vi "VisualizeStatus.vi"(10 "ModuleList":string[](array[string])=["Sync", "FGen", "Digitizer", "Sensor", "Analysis", "Scope", "AcPwr"]) -> ()   [LabVIEW 2018, in "Visualization.lvlib" / "VisualizeStatus.lvclass"]
uses:
  VisualizeStatus.lvclass
  <vilib>/event_ctls.llb/usereventprio.ctl
  VisualizeBase/VisualizeBase_class/Requests/clUserEventType.ctl
  <vilib>/Utility/error.llb/Error Cluster From Error Code.vi
  <vilib>/ErrorRing/Error Ring.xnode
  VisualizeBase/VisualizeBase_class/VisualizeBase.lvclass
  <userlib>/NIST/NISTErrorLib/NISTErrorLib.lvlib
  Sync/SyncModule/SyncModule.lvlib
  Digitizer/DigitizerModule/DigitizerModule.lvlib
  FGen/FgenModule/FgenModule.lvlib
  BusClass/Bus.lvclass
  Sensor/SensorModule/SensorModule.lvlib
  Analysis/AnalysisModule/AnalysisModule.lvlib
  Scope/ScopeModule/ScopeModule.lvlib
panel:
  out "Status Message":string
  in  "btnReset":bool
  in  "btnClear":bool
  in  "QueName":string="BaseVisQue"
  out "ErrorArray":errorcluster[](array[cluster])
  in  "btnStop":bool
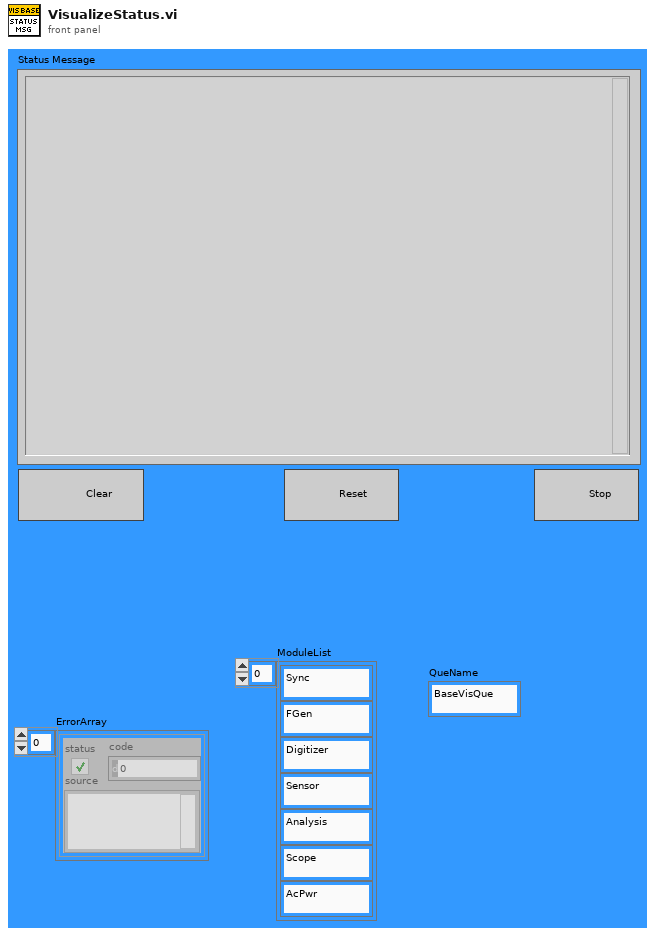
[diagram p1: front panel]
types:
  T1 = typedef "SyncModule.lvlib/clBroadcastEvents.ctl" = cluster{"DidInit":refnum<user-event>, "StatusUpdate":refnum<user-event>, "ErrorReport":refnum<user-event>, "DidStop":refnum<user-event>, "PathToINI":refnum<user-event>, "TriggerTime":refnum<user-event>, "LockStatus":refnum<user-event>, "Info":refnum<user-event>, "ClockProperties":refnum<user-event>}
  T2 = typedef "FgenModule.lvlib/clBroadcastEvents.ctl" = cluster{"DidInit":refnum<user-event>, "StatusUpdate":refnum<user-event>, "ErrorReport":refnum<user-event>, "DidStop":refnum<user-event>, "PathToINI":refnum<user-event>, "Channels":refnum<user-event>, "Function":refnum<user-event>, "Waveforms":refnum<user-event>, "Triggers":refnum<user-event>, "FunctionParams":refnum<user-event>, "FunctionArbs":refnum<user-event>, "FunctionSampleRate":refnum<user-event>}
  T3 = typedef "ScopeModule.lvlib/clBroadcastEvents.ctl" = cluster{"DidInit":refnum<user-event>, "StatusUpdate":refnum<user-event>, "ErrorReport":refnum<user-event>, "DidStop":refnum<user-event>, "PathToINI":refnum<user-event>, "Handle":refnum<user-event>, "Model":refnum<user-event>, "Channels":refnum<user-event>, "Acquisition":refnum<user-event>, "Trigger":refnum<user-event>, "ExtAcquisition":refnum<user-event>, "Waveform":refnum<user-event>}
  T4 = typedef "DigitizerModule.lvlib/clBroadcastEvents.ctl" = cluster{"DidInit":refnum<user-event>, "StatusUpdate":refnum<user-event>, "ErrorReport":refnum<user-event>, "DidStop":refnum<user-event>, "PathToINI":refnum<user-event>, "Channels":refnum<user-event>, "Acq":refnum<user-event>, "Trigger":refnum<user-event>, "Waveforms":refnum<user-event>}
  T5 = typedef "SensorModule.lvlib/clBroadcastEvents.ctl" = cluster{"DidInit":refnum<user-event>, "StatusUpdate":refnum<user-event>, "ErrorReport":refnum<user-event>, "DidStop":refnum<user-event>, "PathToINI":refnum<user-event>, "SensorReport":refnum<user-event>, "SensorConfig":refnum<user-event>}
  T6 = typedef "AnalysisModule.lvlib/clBroadcastEvents.ctl" = cluster{"DidInit":refnum<user-event>, "StatusUpdate":refnum<user-event>, "ErrorReport":refnum<user-event>, "DidStop":refnum<user-event>, "PathToINI":refnum<user-event>, "Config":refnum<user-event>, "ResultReport":refnum<user-event>, "FunctionClass":refnum<user-event>, "State":refnum<user-event>, "FunctionParams":refnum<user-event>}
  T7 = typedef "clBroadcastEvents.ctl" = cluster{"DidInit":refnum<user-event>, "StatusUpdate":refnum<user-event>, "ErrorReport":refnum<user-event>, "DidStop":refnum<user-event>, "PathToINI":refnum<user-event>, "Measurements":refnum<user-event>, "LoadConfigFile":refnum<user-event>, "GetSettings":refnum<user-event>, "SetSettings":refnum<user-event>, "GetType&ID":refnum<user-event>, "GotSettings":refnum<user-event>}
  T8 = cluster{"StatusUpdate":refnum<user-event>, "ErrorReport":refnum<user-event>}
  T9 = typedef "Visualization.lvlib/VisualizeBase.lvclass/clRequestEvents.ctl" = cluster{"StopRequest":refnum<user-event>, "ResetRequest":refnum<user-event>}
  T10 = typedef "usereventprio.ctl" = enum32{"high priority", "normal priority"}
  T11 = typedef "Visualization.lvlib/VisualizeBase.lvclass/clUserEventType.ctl" = cluster{"BusIndex":i8, "Data":variant}
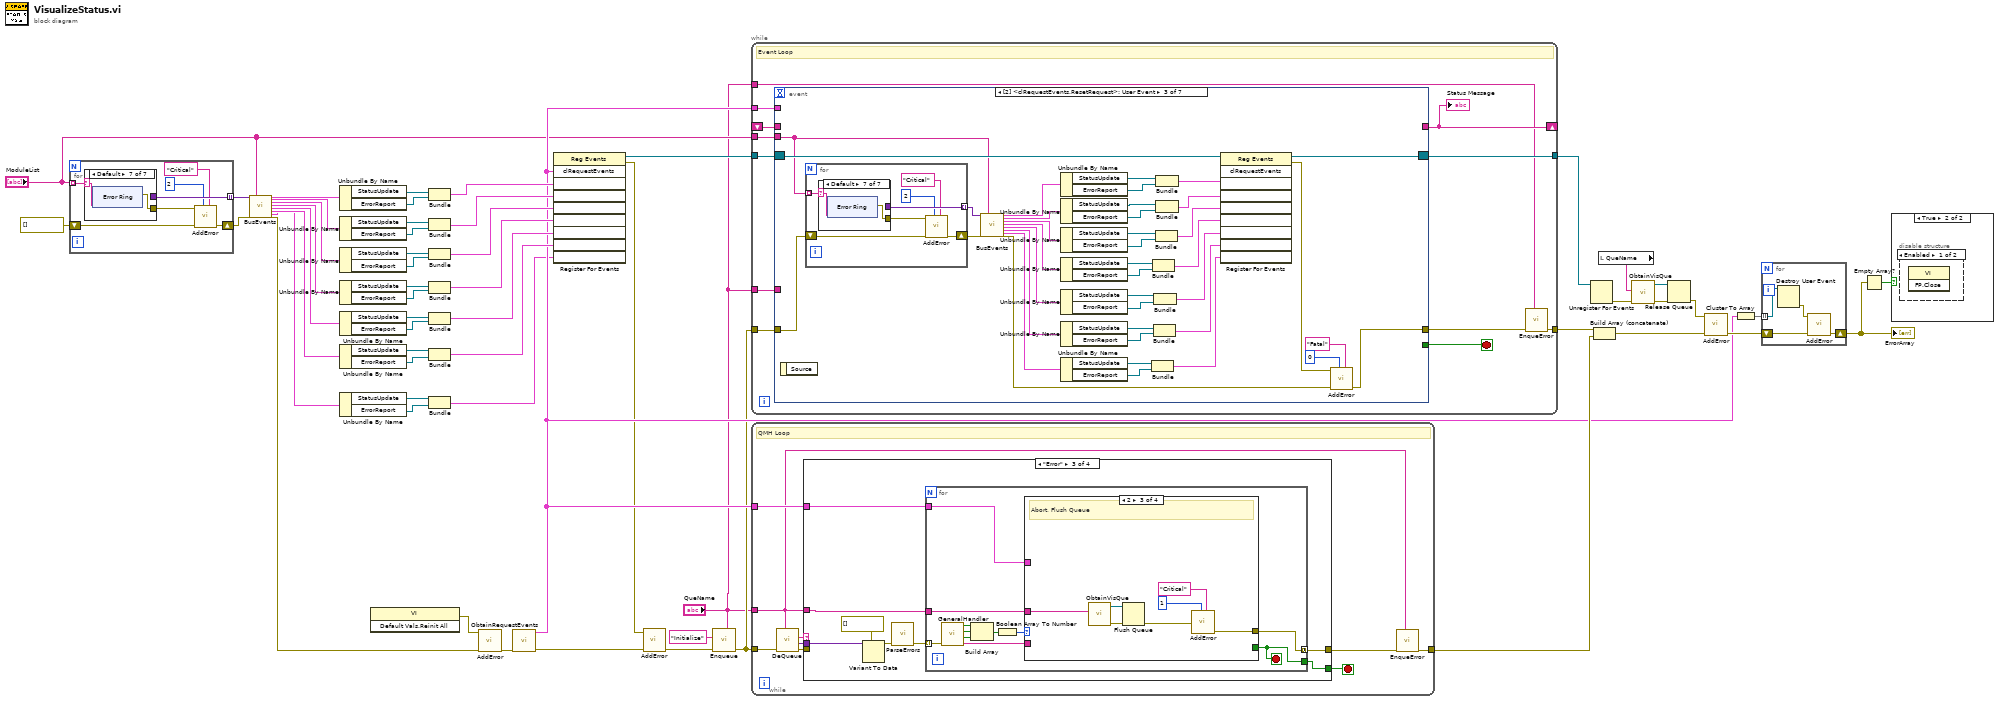
[diagram p0: block diagram]
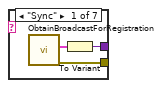
[diagram p2: hidden frame]
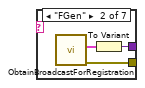
[diagram p3: hidden frame]
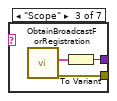
[diagram p4: hidden frame]
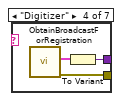
[diagram p5: hidden frame]
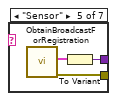
[diagram p6: hidden frame]
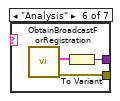
[diagram p7: hidden frame]
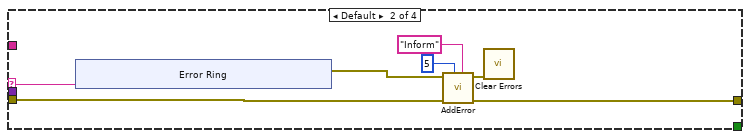
[diagram p9: hidden frame]
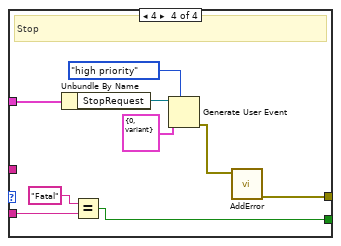
[diagram p12: hidden frame]
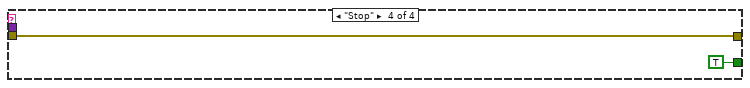
[diagram p13: hidden frame]
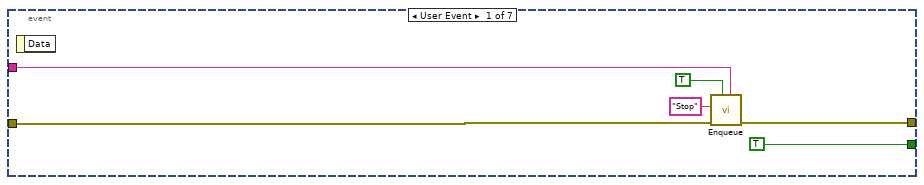
[diagram p14: hidden frame]
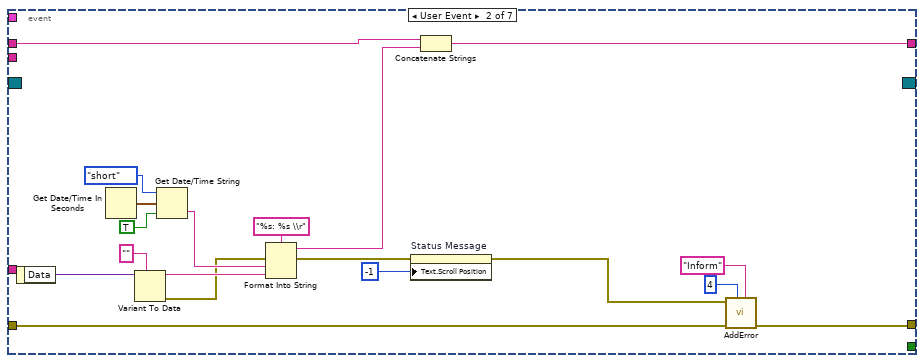
[diagram p15: hidden frame]
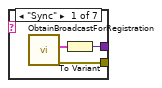
[diagram p16: hidden frame]
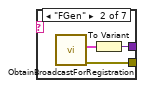
[diagram p17: hidden frame]
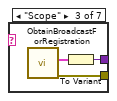
[diagram p18: hidden frame]
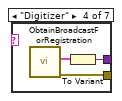
[diagram p19: hidden frame]
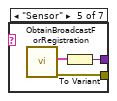
[diagram p20: hidden frame]
diagram:
  n1 = for {
    shift-right: [w62] -> w22
    shift-left: errorcluster[] [] ("ErrorArray") -> [w61]
    tunnel: [w60] -> w23 mode=indexing
    tunnel: "ModuleList" -> [w57] mode=indexing
    n2 = case shown="Default" w57 {
      selector: w57 -> [_ _ _ _ _ _ w82]
      tunnel: [w65 w68 w70 w74 w77 w80 _] -> w60
      tunnel: [w64 w69 w72 w75 w78 w81 w83] -> w63
      frame "Sync" {
        n3 = call "ObtainBroadcastForRegistration.vi"() -> ("error out"=w64:errorcluster, "SyncBroadcastEvents"=w66:T1)  [unwired: 10 in]
        n4 = To Variant(anything=w66) -> (Variant=w65:variant)
      }
      frame "FGen" {
        n5 = call "ObtainBroadcastForRegistration.vi"() -> ("error out"=w69:errorcluster, "clBroadcastEvents"=w67:T2)  [unwired: 10 in]
        n6 = To Variant(anything=w67) -> (Variant=w68:variant)
      }
      frame "Scope" {
        n7 = call "ObtainBroadcastForRegistration.vi"() -> ("error out"=w72:errorcluster, "clBroadcastEvents"=w71:T3)  [unwired: 10 in]
        n8 = To Variant(anything=w71) -> (Variant=w70:variant)
      }
      frame "Digitizer" {
        n9 = call "ObtainBroadcastForRegistration.vi"() -> ("error out"=w75:errorcluster, "clDigitizerBdcstEvents"=w73:T4)  [unwired: 10 in]
        n10 = To Variant(anything=w73) -> (Variant=w74:variant)
      }
      frame "Sensor" {
        n11 = call "ObtainBroadcastForRegistration.vi"() -> ("error out"=w78:errorcluster, "SensorBdcstEvents"=w76:T5)  [unwired: 10 in]
        n12 = To Variant(anything=w76) -> (Variant=w77:variant)
      }
      frame "Analysis" {
        n13 = call "ObtainBroadcastForRegistration.vi"() -> ("error out"=w81:errorcluster, "AnalysisBroadcastEvents"=w79:T6)  [unwired: 10 in]
        n14 = To Variant(anything=w79) -> (Variant=w80:variant)
      }
      frame Default {
        n15 = xnode "Error Ring"("parameter 0"=w82) -> ("error out"=w83:errorcluster)
      }
    }
    n16 = call <userlib>:"AddError.vi"("Severity"="Critical", "Priority"=u8 2, "ErrorArray"=w61, "error in (no error)"=w63) -> ("ErrorArray"=w62:errorcluster[])  [unwired: 6 in, 1 out]
  }
  n17 = call "BusEvents.vi"("EventArray"=w23, "Error in"=w22, "ModuleList"="ModuleList") -> ("SyncEvts"=w32:T1, "FGenEvts"=w31:T2, "DigitizerEvts"=w30:T4, "AnalysisBroadcastEvents"=w25:T6, "SensorBdcstEvents"=w24:T5, "ScopeBdcstEvents"=w16:T3, "clAcPwrEvents"=w5:T7, "Error out"=w6:errorcluster[])  [unwired: 16 in, 1 out]
  n18 = Unbundle By Name(w32) -> ("StatusUpdate"=w39:refnum<user-event>, "ErrorReport"=w38:refnum<user-event>)
  n19 = Unbundle By Name(w31) -> ("StatusUpdate"=w37:refnum<user-event>, "ErrorReport"=w36:refnum<user-event>)
  n20 = Unbundle By Name(w30) -> ("StatusUpdate"=w35:refnum<user-event>, "ErrorReport"=w34:refnum<user-event>)
  n21 = Unbundle By Name(w25) -> ("StatusUpdate"=w28:refnum<user-event>, "ErrorReport"=w29:refnum<user-event>)
  n22 = Unbundle By Name(w24) -> ("StatusUpdate"=w27:refnum<user-event>, "ErrorReport"=w26:refnum<user-event>)
  n23 = Unbundle By Name(w16) -> ("StatusUpdate"=w18:refnum<user-event>, "ErrorReport"=w17:refnum<user-event>)
  n24 = Unbundle By Name(w5) -> ("StatusUpdate"=w8:refnum<user-event>, "ErrorReport"=w9:refnum<user-event>)
  n25 = invoke class="VI" method="Default Vals.Reinit All"() -> (error out=w55:errorcluster)  [unwired: 3 in, 2 out]
  n26 = Bundle("StatusUpdate"=w39, "ErrorReport"=w38) -> (w15:T8)  [unwired: 1 in]
  n27 = Bundle("StatusUpdate"=w37, "ErrorReport"=w36) -> (w13:T8)  [unwired: 1 in]
  n28 = Bundle("StatusUpdate"=w35, "ErrorReport"=w34) -> (w14:T8)  [unwired: 1 in]
  n29 = Bundle("StatusUpdate"=w28, "ErrorReport"=w29) -> (w12:T8)  [unwired: 1 in]
  n30 = Bundle("StatusUpdate"=w27, "ErrorReport"=w26) -> (w20:T8)  [unwired: 1 in]
  n31 = Bundle("StatusUpdate"=w18, "ErrorReport"=w17) -> (w19:T8)  [unwired: 1 in]
  n32 = Bundle("StatusUpdate"=w8, "ErrorReport"=w9) -> (w7:T8)  [unwired: 1 in]
  n33 = call <userlib>:"AddError.vi"("ErrorArray"=w6, "error in (no error)"=w55) -> ("ErrorArray"=w54:errorcluster[])  [unwired: 8 in, 1 out]
  n34 = call "ObtainRequestEvents.vi"("Error"=w54) -> ("Error"=w53:errorcluster[], "clRequestEvents"=w11:T9)  [unwired: 9 in]
  n35 = register-events(w11, w15, w13, w14, w12, w20, w19, w7) -> (reference out=w21:refnum<event-registration>, error out=w10:errorcluster)  [unwired: 2 in]
  n36 = call <userlib>:"AddError.vi"("ErrorArray"=w53, "error in (no error)"=w10) -> ("ErrorArray"=w33:errorcluster[])  [unwired: 8 in, 1 out]
  n37 = call "Enqueue.vi"("QueName"="QueName", "Error"=w33, "Message"="Initialize") -> ("Error"=w3:errorcluster[])  [unwired: 8 in]
  n38 = while {
    tunnel: w21 -> [w102]
    tunnel: [w99] -> w50
    tunnel: [w98] -> w52
    tunnel: w11 -> [w97]
    shift-right: [w93] -> _
    shift-left: _ -> [w96]
    tunnel: w3 -> [w95]
    tunnel: "ModuleList" -> [w94]
    tunnel: "QueName" -> [w92]
    tunnel: "QueName" -> [w91]
    stop <- w101 stop-if-true
    # "Event Loop"
    n39 = event shown="[2] <clRequestEvents.ResetRequest>: User Event" {
      selector: w102 -> [_ _ w143 _ _ _ _]
      dyn-events: [_ _ w145 _ _ _ _] -> w98
      timeout: _ -> [_ _ _ _ _ _ _]
      tunnel: [TRUE _ _ _ _ _ _] -> w101
      tunnel: [w107 w118 w160 w210 _ w228 w233] -> w100
      tunnel: w97 -> [_ _ _ _ _ w223 w232]
      tunnel: [_ w114 _ w205 "" _ _] -> w93
      tunnel: w96 -> [_ w113 _ w204 _ _ _]
      tunnel: w95 -> [w103 w112 w138 w201 _ w222 w231]
      tunnel: w94 -> [_ _ w137 _ _ _ _]
      tunnel: w91 -> [w104 _ _ _ _ _ _]
      event User Event {
        n40 = event-data() -> ()  [unwired: 1 in, 1 out]
        n41 = call "Enqueue.vi"("QueName"=w104, "Priority? (F)"=TRUE, "Error"=w103, "Message"="Stop") -> ("Error"=w107:errorcluster[])  [unwired: 7 in]
      }
      event User Event {
        n42 = event-data() -> ("Data"=w124:variant)  [unwired: 1 in]
        n43 = Get Date/Time In Seconds() -> (seconds since 1Jan1904=w127:timestamp)
        n44 = Variant To Data(type="", Variant=w124) -> (data=w120:string, error out=w119:errorcluster)  [unwired: 1 in]
        n45 = Get Date/Time String(date format (0)=enum16{"short", "long", "abbreviated"}."short", seconds (now)=w127, want seconds? (F)=TRUE) -> (time string=w121:string)  [unwired: 1 out]
        n46 = Format Into String(format string="%s: %s \\r", error in=w119, w121, w120) -> (resulting string=w115:string, error out=w111:errorcluster)  [unwired: 1 in]
        n47 = property on="Status Message" class="Str"(error in=w111, "Text.Scroll Position"=-1) -> (error out=w110:errorcluster)  [unwired: 1 in, 1 out]
        n48 = Concatenate Strings(w113, w115) -> (w114:string)
        n49 = call <userlib>:"AddError.vi"("Severity"="Inform", "Priority"=u8 4, "ErrorArray"=w112, "error in (no error)"=w110) -> ("ErrorArray"=w118:errorcluster[])  [unwired: 6 in, 1 out]
      }
      event User Event {
        n50 = event-data() -> ()  [unwired: 1 in, 1 out]
        n51 = for {
          shift-right: [w172] -> w148
          shift-left: w138 -> [w171]
          tunnel: [w170] -> w146 mode=indexing
          tunnel: w137 -> [w167] mode=indexing
          n52 = case shown="Default" w167 {
            selector: w167 -> [_ _ _ _ _ _ w192]
            tunnel: [w175 w178 w182 w184 w187 w190 _] -> w170
            tunnel: [w174 w179 w181 w185 w188 w191 w193] -> w173
            frame "Sync" {
              n53 = call "ObtainBroadcastForRegistration.vi"() -> ("error out"=w174:errorcluster, "SyncBroadcastEvents"=w176:T1)  [unwired: 10 in]
              n54 = To Variant(anything=w176) -> (Variant=w175:variant)
            }
            frame "FGen" {
              n55 = call "ObtainBroadcastForRegistration.vi"() -> ("error out"=w179:errorcluster, "clBroadcastEvents"=w177:T2)  [unwired: 10 in]
              n56 = To Variant(anything=w177) -> (Variant=w178:variant)
            }
            frame "Scope" {
              n57 = call "ObtainBroadcastForRegistration.vi"() -> ("error out"=w181:errorcluster, "clBroadcastEvents"=w180:T3)  [unwired: 10 in]
              n58 = To Variant(anything=w180) -> (Variant=w182:variant)
            }
            frame "Digitizer" {
              n59 = call "ObtainBroadcastForRegistration.vi"() -> ("error out"=w185:errorcluster, "clDigitizerBdcstEvents"=w183:T4)  [unwired: 10 in]
              n60 = To Variant(anything=w183) -> (Variant=w184:variant)
            }
            frame "Sensor" {
              n61 = call "ObtainBroadcastForRegistration.vi"() -> ("error out"=w188:errorcluster, "SensorBdcstEvents"=w186:T5)  [unwired: 10 in]
              n62 = To Variant(anything=w186) -> (Variant=w187:variant)
            }
            frame "Analysis" {
              n63 = call "ObtainBroadcastForRegistration.vi"() -> ("error out"=w191:errorcluster, "AnalysisBroadcastEvents"=w189:T6)  [unwired: 10 in]
              n64 = To Variant(anything=w189) -> (Variant=w190:variant)
            }
            frame Default {
              n65 = xnode "Error Ring"("parameter 0"=w192) -> ("error out"=w193:errorcluster)
            }
          }
          n66 = call <userlib>:"AddError.vi"("Severity"="Critical", "Priority"=u8 2, "ErrorArray"=w171, "error in (no error)"=w173) -> ("ErrorArray"=w172:errorcluster[])  [unwired: 6 in, 1 out]
        }
        n67 = call "BusEvents.vi"("EventArray"=w146, "Error in"=w148, "ModuleList"=w137) -> ("SyncEvts"=w155:T1, "FGenEvts"=w154:T2, "DigitizerEvts"=w153:T4, "AnalysisBroadcastEvents"=w152:T6, "SensorBdcstEvents"=w151:T5, "ScopeBdcstEvents"=w140:T3, "clAcPwrEvents"=w139:T7, "Error out"=w147:errorcluster[])  [unwired: 16 in, 1 out]
        n68 = Unbundle By Name(w155) -> ("StatusUpdate"=w161:refnum<user-event>, "ErrorReport"=w162:refnum<user-event>)
        n69 = Unbundle By Name(w154) -> ("StatusUpdate"=w163:refnum<user-event>, "ErrorReport"=w164:refnum<user-event>)
        n70 = Unbundle By Name(w153) -> ("StatusUpdate"=w165:refnum<user-event>, "ErrorReport"=w166:refnum<user-event>)
        n71 = Unbundle By Name(w152) -> ("StatusUpdate"=w150:refnum<user-event>, "ErrorReport"=w157:refnum<user-event>)
        n72 = Unbundle By Name(w151) -> ("StatusUpdate"=w149:refnum<user-event>, "ErrorReport"=w156:refnum<user-event>)
        n73 = Unbundle By Name(w140) -> ("StatusUpdate"=w142:refnum<user-event>, "ErrorReport"=w141:refnum<user-event>)
        n74 = Unbundle By Name(w139) -> ("StatusUpdate"=w136:refnum<user-event>, "ErrorReport"=w135:refnum<user-event>)
        n75 = Bundle("StatusUpdate"=w136, "ErrorReport"=w135) -> (w128:T8)  [unwired: 1 in]
        n76 = Bundle("StatusUpdate"=w150, "ErrorReport"=w157) -> (w131:T8)  [unwired: 1 in]
        n77 = Bundle("StatusUpdate"=w142, "ErrorReport"=w141) -> (w129:T8)  [unwired: 1 in]
        n78 = Bundle("StatusUpdate"=w149, "ErrorReport"=w156) -> (w130:T8)  [unwired: 1 in]
        n79 = Bundle("StatusUpdate"=w165, "ErrorReport"=w166) -> (w132:T8)  [unwired: 1 in]
        n80 = Bundle("StatusUpdate"=w161, "ErrorReport"=w162) -> (w134:T8)  [unwired: 1 in]
        n81 = Bundle("StatusUpdate"=w163, "ErrorReport"=w164) -> (w133:T8)  [unwired: 1 in]
        n82 = register-events(reference=w143, w134, w133, w132, w131, w130, w129, w128) -> (reference out=w145:refnum<event-registration>, error out=w144:errorcluster)  [unwired: 2 in]
        n83 = call <userlib>:"AddError.vi"("Severity"="Fatal", "Priority"=u8 0, "ErrorArray"=w147, "error in (no error)"=w144) -> ("ErrorArray"=w160:errorcluster[])  [unwired: 6 in, 1 out]
      }
      event User Event {
        n84 = event-data() -> ("Data"=w217:variant)  [unwired: 1 in]
        n85 = Get Date/Time In Seconds() -> (seconds since 1Jan1904=w220:timestamp)
        n86 = Variant To Data(type=errorcluster {"status"=FALSE, "code"=0, "source"=""} ("error constant"), Variant=w217) -> (data=w214:errorcluster, error out=w213:errorcluster)  [unwired: 1 in]
        n87 = Get Date/Time String(date format (0)=enum16{"short", "long", "abbreviated"}."short", seconds (now)=w220, want seconds? (F)=TRUE) -> (time string=w215:string)  [unwired: 1 out]
        n88 = Unbundle By Name(w214) -> ("source"=w202:string)
        n89 = Format Into String(format string="%s: %s \\r", error in=w213, w215, w202) -> (resulting string=w206:string, error out=w212:errorcluster)  [unwired: 1 in]
        n90 = property on="Status Message" class="Str"(error in=w212, "Text.Scroll Position"=-1) -> (error out=w209:errorcluster)  [unwired: 1 in, 1 out]
        n91 = Concatenate Strings(w204, w206) -> (w205:string)
        n92 = call <userlib>:"AddError.vi"("Severity"="Inform", "Priority"=u8 4, "ErrorArray"=w201, "error in (no error)"=w209) -> ("ErrorArray"=w210:errorcluster[])  [unwired: 6 in, 1 out]
      }
      event "btnClear": Value Change {
        n93 = event-data() -> ()  [unwired: 1 in, 1 out]
      }
      event "btnStop": Value Change {
        n94 = event-data() -> ()  [unwired: 1 in, 1 out]
        n95 = Unbundle By Name(w223) -> ("StopRequest"=w229:refnum<user-event>)
        n96 = Generate User Event(priority (normal)=usereventprio."high priority", user event=w229, event data cluster=T11 {"BusIndex"=0, "Data"=variant} ("event data")) -> (error out=w230:errorcluster)  [unwired: 1 in, 1 out]
        n97 = call <userlib>:"AddError.vi"("Severity"="Fatal" ("String"), "Priority"=u8 0, "ErrorArray"=w222, "error in (no error)"=w230) -> ("ErrorArray"=w228:errorcluster[])  [unwired: 6 in, 1 out]
      }
      event "btnReset": Value Change {
        n98 = event-data() -> ()  [unwired: 1 in, 1 out]
        n99 = Unbundle By Name(w232) -> ("ResetRequest"=w234:refnum<user-event>)
        n100 = Generate User Event(priority (normal)=usereventprio."high priority", user event=w234, event data cluster=T11 {"BusIndex"=0, "Data"=variant} ("event data")) -> (error out=w237:errorcluster)  [unwired: 1 in, 1 out]
        n101 = call <userlib>:"AddError.vi"("Severity"="Fatal", "Priority"=u8 0, "ErrorArray"=w231, "error in (no error)"=w237) -> ("ErrorArray"=w233:errorcluster[])  [unwired: 6 in, 1 out]
      }
    }
    "Status Message" <- w93
    n102 = call "EnqueError.vi"("QueName"=w92, "Error"=w100) -> ("Error"=w99:errorcluster[])  [unwired: 9 in]
  }
  n103 = while {
    tunnel: w3 -> [w248]
    tunnel: [w242] -> w49
    tunnel: w11 -> [w241]
    tunnel: "QueName" -> [w240]
    stop <- w243 stop-if-true
    # "QMH Loop"
    n104 = call "DeQueue.vi"("QueName"=w240, "Error"=w248) -> ("Error"=w245:errorcluster[], "Data"=w246:variant, "Message"=w247:string)  [unwired: 7 in]
    n105 = case shown="\"Error\"" w247 {
      selector: w247 -> [_ w256 _ _]
      tunnel: w246 -> [_ _ w271 _]
      tunnel: w245 -> [w249 w254 _ w299]
      tunnel: [w249 w253 w267 w299] -> w244
      tunnel: [_ _ w266 TRUE] -> w243
      tunnel: w241 -> [_ _ w265 _]
      tunnel: w240 -> [_ _ w264 _]
      frame "Initialize" {
      }
      frame Default {
        n106 = xnode "Error Ring"("parameter 0"=w256) -> ("error out"=w255:errorcluster)
        n107 = call <userlib>:"AddError.vi"("Severity"="Inform" ("String"), "Priority"=u8 5, "ErrorArray"=w254, "error in (no error)"=w255) -> ("ErrorArray"=w253:errorcluster[], "error out"=w252:errorcluster)  [unwired: 6 in]
        n108 = call <vilib>:"Clear Errors.vi"("error in (no error)"=w252) -> ()  [unwired: 5 in, 2 out]
      }
      frame "Error" {
        n109 = Variant To Data(type=errorcluster[] [], Variant=w271) -> (data=w269:errorcluster[])  [unwired: 1 in, 1 out]
        n110 = call <userlib>:"ParseErrors.vi"("ErrorArray"=w269) -> ("ErrorArray"=w268:errorcluster[])  [unwired: 8 in, 2 out]
        n111 = for {
          tunnel: w268 -> [w282] mode=indexing
          tunnel: [w276] -> w267 mode=concatenating
          tunnel: [w274] -> w266
          tunnel: w265 -> [w273]
          tunnel: w264 -> [w272]
          stop <- w274 stop-if-true
          n112 = call <userlib>:"GeneralHandler.vi"("error in (no error)"=w282) -> ("Severity"=w275:string, "Stop"=w279:bool, "Abort"=w280:bool, "Continue"=w281:bool)  [unwired: 7 in]
          n113 = Build Array(w281, w280, w279) -> (w278:bool[])
          n114 = Boolean Array To Number(Boolean array=w278) -> (number=w277:u32)
          n115 = case shown="2" w277 {
            tunnel: [_ _ w287 w297] -> w276
            tunnel: w275 -> [_ _ _ w293]
            tunnel: [_ _ _ w291] -> w274
            tunnel: w273 -> [_ _ _ w290]
            tunnel: w272 -> [_ _ w283 _]
            frame 0, Default {
              # "No Dialog"
            }
            frame 1 {
              # "Continue"
            }
            frame 2 {
              # "Abort, Flush Queue"
              n116 = call "ObtainVisQue.vi"("QueName"=w283) -> ("error out"=w289:errorcluster, "queue out"=w288:refnum<queue>)  [unwired: 9 in]
              n117 = Flush Queue(queue=w288, error in (no error)=w289) -> (error out=w286:errorcluster)  [unwired: 2 out]
              n118 = call <userlib>:"AddError.vi"("Severity"="Critical" ("String"), "Priority"=u8 1, "error in (no error)"=w286) -> ("ErrorArray"=w287:errorcluster[])  [unwired: 7 in, 1 out]
            }
            frame 4 {
              # "Stop"
              n119 = Unbundle By Name(w290) -> ("StopRequest"=w298:refnum<user-event>)
              n120 = Equal?(x="Fatal", y=w293) -> (x = y?=w291:bool)
              n121 = Generate User Event(priority (normal)=usereventprio."high priority", user event=w298, event data cluster=T11 {"BusIndex"=0, "Data"=variant} ("event data")) -> (error out=w296:errorcluster)  [unwired: 1 in, 1 out]
              n122 = call <userlib>:"AddError.vi"("error in (no error)"=w296) -> ("ErrorArray"=w297:errorcluster[])  [unwired: 9 in, 1 out]
            }
          }
        }
      }
      frame "Stop" {
      }
    }
    n123 = call "EnqueError.vi"("QueName"=w240, "Error"=w244) -> ("Error"=w242:errorcluster[])  [unwired: 9 in]
  }
  n124 = Unregister For Events(event registration refnum=w52) -> (error out=w48:errorcluster)  [unwired: 1 in]
  n125 = Build Array (concatenate)(w50, w49) -> (w46:errorcluster[])
  n126 = local read "QueName"() -> (w47:string)
  n127 = call "ObtainVisQue.vi"("error in (no error)"=w48, "QueName"=w47) -> ("error out"=w45:errorcluster, "queue out"=w44:refnum<queue>)  [unwired: 8 in]
  n128 = Release Queue(queue=w44, error in (no error)=w45) -> (error out=w43:errorcluster)  [unwired: 1 in, 2 out]
  n129 = call <userlib>:"AddError.vi"("ErrorArray"=w46, "error in (no error)"=w43) -> ("ErrorArray"=w42:errorcluster[])  [unwired: 8 in, 1 out]
  n130 = Cluster To Array(cluster=w11) -> (array=w51:refnum<user-event>[])
  n131 = for {
    tunnel: w51 -> [w304] mode=indexing
    shift-right: [w303] -> w41
    shift-left: w42 -> [w302]
    n132 = Destroy User Event(user event=w304) -> (error out=w301:errorcluster)  [unwired: 1 in]
    n133 = call <userlib>:"AddError.vi"("ErrorArray"=w302, "error in (no error)"=w301) -> ("ErrorArray"=w303:errorcluster[])  [unwired: 8 in, 1 out]
  }
  "ErrorArray" <- w41
  n134 = Empty Array?(array=w41) -> (empty?=w40:bool)
  n135 = case shown="True" w40 {
    frame False {
    }
    frame True {
      n136 = disable-structure shown="Enabled" {
        frame Enabled {
          n137 = invoke class="VI" method="FP.Close"() -> ()  [unwired: 3 in, 3 out]
        }
        frame Disabled {
        }
      }
    }
  }
